vi "Load Spectrum.vi"() -> (2 "Intensity":dbl[](array[numeric]), 3 "Wavelength":dbl[](array[numeric]), 5 "Graph Cluster":cluster{dbl[], dbl[]})   [LabVIEW 2010]
uses:
  <vilib>/Utility/file.llb/Read From Spreadsheet File (DBL).vi
panel:
  # "Imports a 2D-array containing WI data.\nW (wavelength/Raman shift) varies over rows."
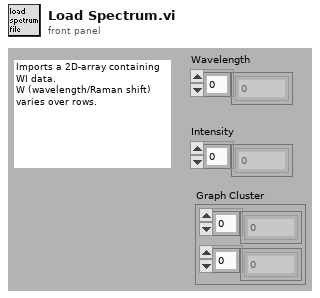
[diagram p1: front panel]
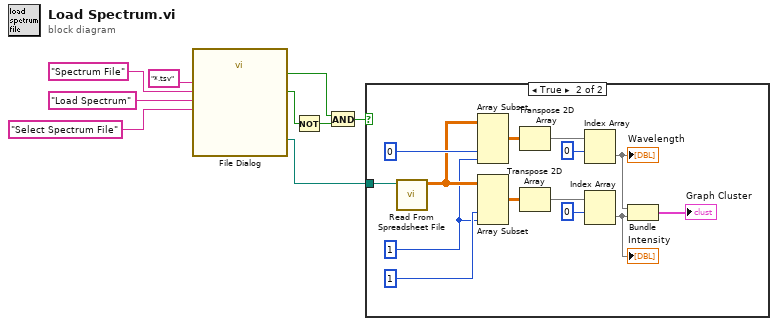
[diagram p0: block diagram]
diagram:
  n1 = call "File Dialog"("prompt"="Select Spectrum File", "button label"="Load Spectrum", "pattern (all files)"="*.tsv", "pattern label"="Spectrum File") -> ("selected path"=w9:path, "exists"=w8:bool, "cancelled"=w6:bool)  [unwired: 8 in, 1 out]
  n2 = Not(x=w6) -> (.not. x?=w7:bool)
  n3 = And(x=w8, y=w7) -> (x .and. y?=w5:bool)
  n4 = case shown="True" w5 {
    tunnel: w9 -> [_ w17]
    frame False {
    }
    frame True {
      w15 = 1 ("Länge")
      n5 = call-poly <vilib>:"Read From Spreadsheet File.vi"("file path (dialog if empty)"=w17) -> ("all rows"=w16:dbl[][])  [unwired: 6 in, 4 out]
      n6 = Array Subset(array=w16, index (col)=0 ("Index"), length (col)=w15) -> (w21:dbl[][])  [unwired: 2 in]
      n7 = Array Subset(array=w16, index (col)=1 ("Index"), length (col)=w15) -> (w19:dbl[][])  [unwired: 2 in]
      n8 = Transpose 2D Array(2D array=w21) -> (transposed array=w20:dbl[][])
      n9 = Transpose 2D Array(2D array=w19) -> (transposed array=w12:dbl[][])
      n10 = Index Array(array=w20, index (row)=0 ("Index")) -> (element=w14:dbl[])  [unwired: 1 in]
      "Wavelength" <- w14
      n11 = Index Array(array=w12, index (row)=0 ("Index")) -> (element=w11:dbl[])  [unwired: 1 in]
      "Intensity" <- w11
      n12 = Bundle(w14, w11) -> (→"Graph Cluster":cluster{dbl[], dbl[]})  [unwired: 1 in]
    }
  }
